vi "iHR550 Correct Center v10.6.2.vi"(1 "Calibration File":path, 2 "Set?":bool=TRUE, 3 "Description":string="1", 4 "Position In (nm)":dbl=897.9988) -> (0 "Position Out (nm)":dbl=897.9988)   [LabVIEW 2010]
uses:
  <vilib>/Utility/config.llb/Read Key (Double).vi
  <vilib>/Utility/config.llb/NI_LVConfig.lvlib
panel:
  out "Error Out":errorcluster
  in  "Error In":errorcluster
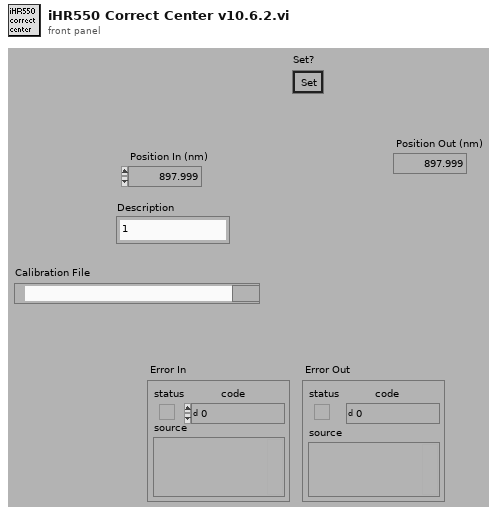
[diagram p1: front panel]
types:
  T1 = typedef "NI_LVConfig.lvlib/Config Data RefNum.ctl" = refnum<k1>
  T2 = cluster{"[0]":dbl, "[1]":dbl, "[2]":dbl, "[3]":dbl}
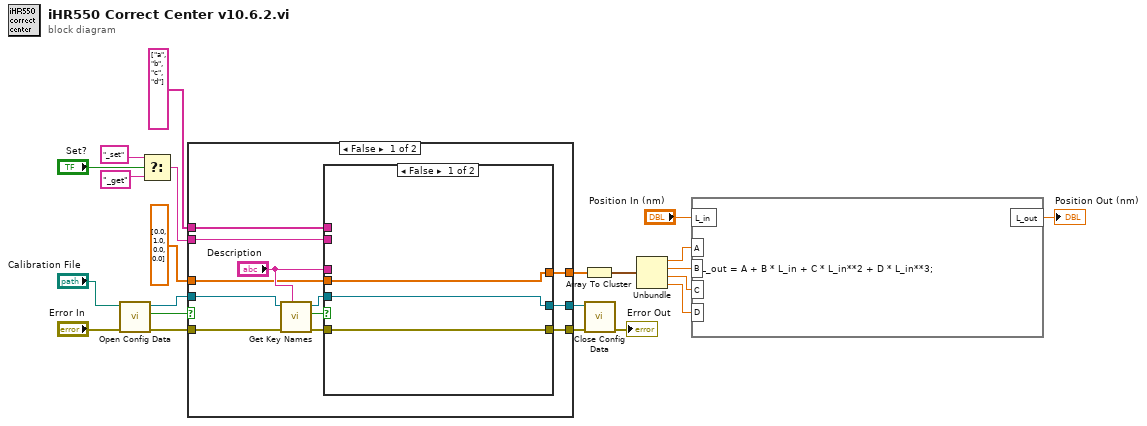
[diagram p0: block diagram]
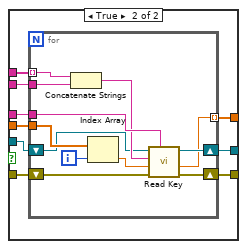
[diagram p2: hidden frame]
diagram:
  n1 = call <vilib>:"Open Config Data.vi"("error in (no error)"="Error In", "configuration file path"="Calibration File") -> ("error out"=w17:errorcluster, "file created?"=w19:bool, "refnum"=w18:T1)  [unwired: 7 in]
  n2 = Select(t="_set", s="Set?", f="_get") -> (s? t:f=w2:string)
  n3 = case shown="False" w19 {
    tunnel: w18 -> [w34 w60]
    tunnel: w17 -> [w33 w61]
    tunnel: [w28 w61] -> w16
    tunnel: [w27 w60] -> w14
    tunnel: [w26 w59] -> w11
    tunnel: dbl[] [0.0, 1.0, 0.0, 0.0] -> [w25 w59]
    tunnel: string[] ["a", "b", "c", "d"] -> [w24 _]
    tunnel: w2 -> [w23 _]
    frame False {
      n4 = call <vilib>:"Get Key Names.vi"("section"="Description", "error in (no error)"=w33, "refnum"=w34) -> ("error out"=w29:errorcluster, "section exists?"=w32:bool, "refnum out"=w31:T1)  [unwired: 5 in, 1 out]
      n5 = case shown="False" w32 {
        tunnel: w31 -> [w37 w40]
        tunnel: "Description" -> [_ w46]
        tunnel: w29 -> [w36 w39]
        tunnel: [w36 w45] -> w28
        tunnel: [w37 w44] -> w27
        tunnel: [w35 w43] -> w26
        tunnel: w25 -> [w35 w42]
        tunnel: w24 -> [_ w41]
        tunnel: w23 -> [_ w38]
        frame False {
        }
        frame True {
          n6 = for {
            tunnel: w46 -> [w58]
            tunnel: w41 -> [w56] mode=indexing
            tunnel: w38 -> [w57]
            tunnel: w42 -> [w51]
            shift-right: [w54] -> w45
            shift-left: w39 -> [w47]
            shift-right: [w53] -> w44
            shift-left: w40 -> [w48]
            tunnel: [w52] -> w43 mode=indexing
            i -> [w49]
            n7 = Concatenate Strings(w56, w57) -> (w55:string)
            n8 = Index Array(array=w51, index=w49) -> (element=w50:dbl)
            n9 = call-poly <vilib>:"Read Key.vi"("section"=w58, "error in (no error)"=w47, "default value"=w50, "key"=w55, "refnum"=w48) -> ("error out"=w54:errorcluster, "value"=w52:dbl, "refnum out"=w53:T1)  [unwired: 3 in, 1 out]
          }
        }
      }
    }
    frame True {
    }
  }
  n10 = Array To Cluster(array=w11) -> (cluster=w10:T2)
  n11 = call <vilib>:"Close Config Data.vi"("error in (no error)"=w16, "refnum"=w14) -> ("error out"=→"Error Out":errorcluster)  [unwired: 8 in, 1 out]
  n12 = Unbundle(w10) -> ("[0]"=w9:dbl, "[1]"=w8:dbl, "[2]"=w7:dbl, "[3]"=w6:dbl)
  n13 = formula code="L_out = A + B * L_in + C * L_in**2 + D * L_in**3;"("L_in"="Position In (nm)", "A"=w9, "B"=w8, "C"=w7, "D"=w6) -> ("L_out"=→"Position Out (nm)":dbl)
